vi "Configure TCP Client Connection.vi"(5 "Connection.TCP":refnum<class "Connection.TCP.lvclass">, 6 "timeout (5000ms)":i32=5000, 8 "error in (no error)":errorcluster, 11 "Authority (localhost:80)":string="localhost:80") -> (0 "error out":errorcluster, 3 "Connection.TCP":refnum<class "Connection.TCP.lvclass">)   [LabVIEW 2013, in "Connection.TCP_GOSPL.lvlib" / "Connection.TCP.lvclass"]
uses:
  Connection.TCP.lvclass
  Connection/Connection.lvclass/Connection.ctl
  Connection/Connection.lvclass
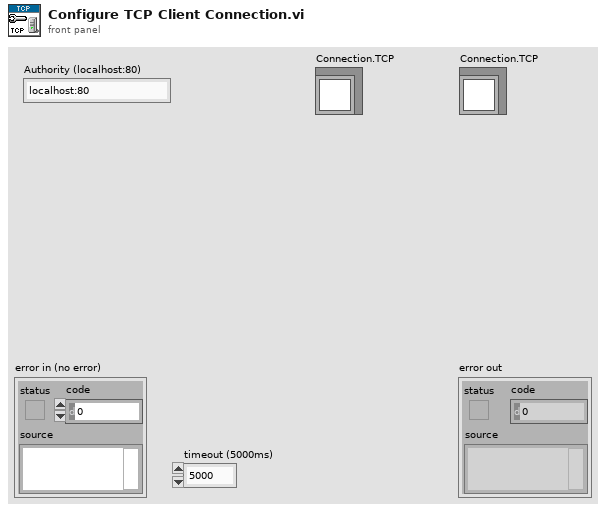
[diagram p1: front panel]
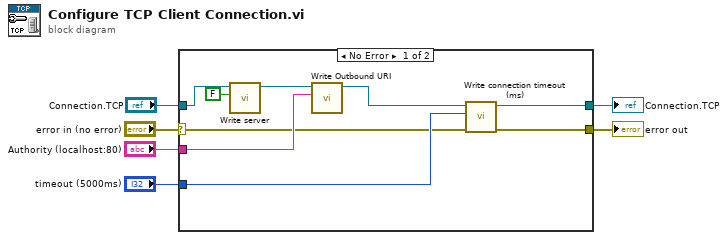
[diagram p0: block diagram]
diagram:
  n1 = case shown="No Error" "error in (no error)" {
    selector: "error in (no error)" -> [w7 w17]
    tunnel: [w13 w17] -> w5
    tunnel: [w14 w16] -> w2
    tunnel: "Authority (localhost:80)" -> [w9 _]
    tunnel: "timeout (5000ms)" -> [w15 _]
    tunnel: "Connection.TCP" -> [w11 w16]
    frame No Error {
      n2 = call "Write server.vi"("server"=FALSE, "Connection in"=w11) -> ("Connection out"=w10:refnum<class "Connection.TCP.lvclass">)  [unwired: 9 in]
      n3 = call "Write Outbound URI.vi"("Outbound URI"=w9, "Connection in"=w10) -> ("Connection out"=w8:refnum<class "Connection.TCP.lvclass">)  [unwired: 9 in]
      n4 = call "Write connection timeout (ms).vi"("error in (no error)"=w7, "connection timeout (ms)"=w15, "Connection in"=w8) -> ("error out"=w13:errorcluster, "Connection out"=w14:refnum<class "Connection.TCP.lvclass">)  [unwired: 7 in]
    }
    frame Error {
    }
  }
  "error out" <- w5
  "Connection.TCP" <- w2
